vi "Listbox-Get Selections.vi"(8 "error in (no error)":errorcluster, 11 "Listbox Ref":refnum<vi>) -> (0 "error out":errorcluster, 3 "Selections":string[](array[string]))   [LabVIEW 2020]
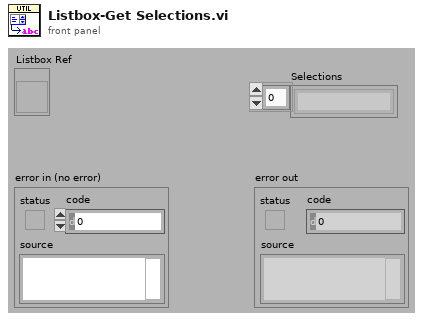
[diagram p1: front panel]
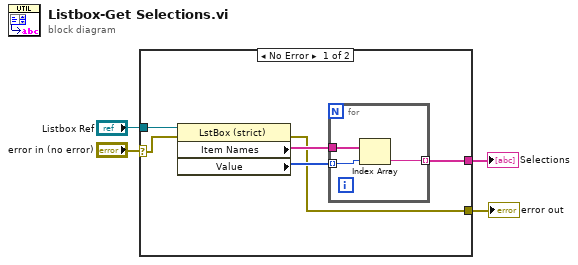
[diagram p0: block diagram]
diagram:
  n1 = case shown="No Error" "error in (no error)" {
    selector: "error in (no error)" -> [w6 w14]
    tunnel: "Listbox Ref" -> [w10 _]
    tunnel: [w7 _] -> w3
    tunnel: [w5 w14] -> w1
    frame No Error {
      n2 = property class="LstBox (strict)"(reference=w10, error in=w6) -> (error out=w5:errorcluster, "Item Names"=w9:string[], "Value"=w8:i32[])  [unwired: 1 out]
      n3 = for {
        tunnel: w9 -> [w13]
        tunnel: w8 -> [w12] mode=indexing
        tunnel: [w11] -> w7 mode=indexing
        n4 = Index Array(array=w13, index=w12) -> (element=w11:string)
      }
    }
    frame Error {
    }
  }
  "error out" <- w1
  "Selections" <- w3
